vi "run_py.vi"(8 "error_in":errorcluster, 11 "preregistraion_data":T1) -> (0 "error_out":errorcluster)   [LabVIEW 2018]
uses:
  controls/preregistration_data.ctl
panel:
  out "mac_db.txt creation progress":i32(slide) scale=0.0..65535.0
  in  "stop":bool
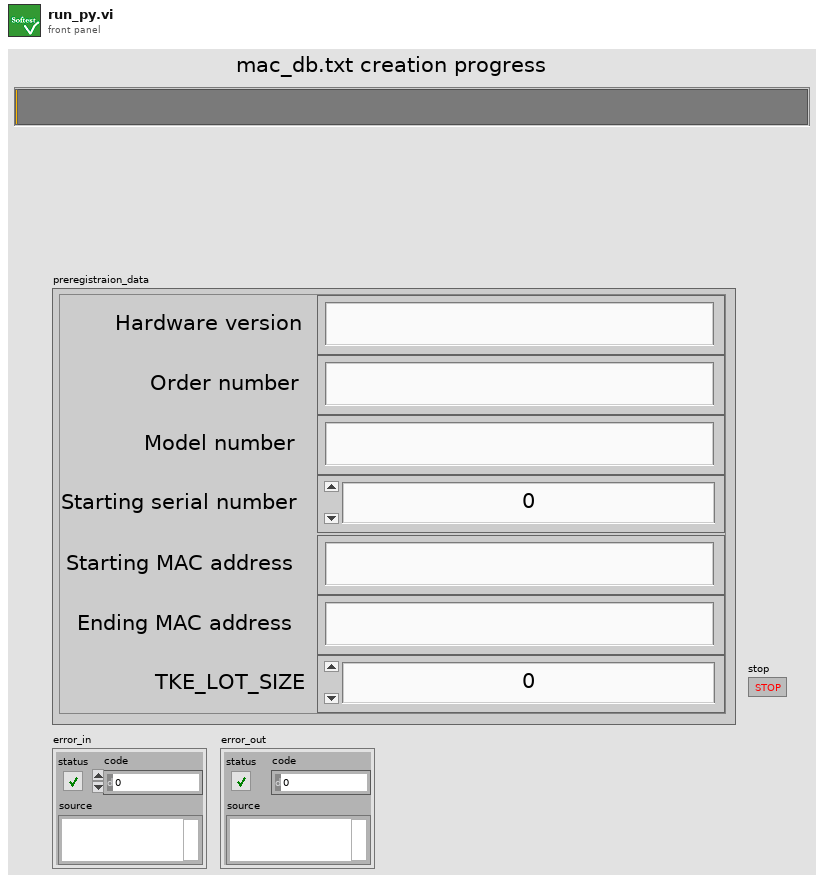
[diagram p1: front panel]
types:
  T1 = typedef "preregistration_data.ctl" = cluster{"Hardware version":string, "Order number":string, "Model number":string, "Starting serial number":i32, "Starting MAC address":string, "Ending MAC address":string, "TKE_LOT_SIZE":i32}
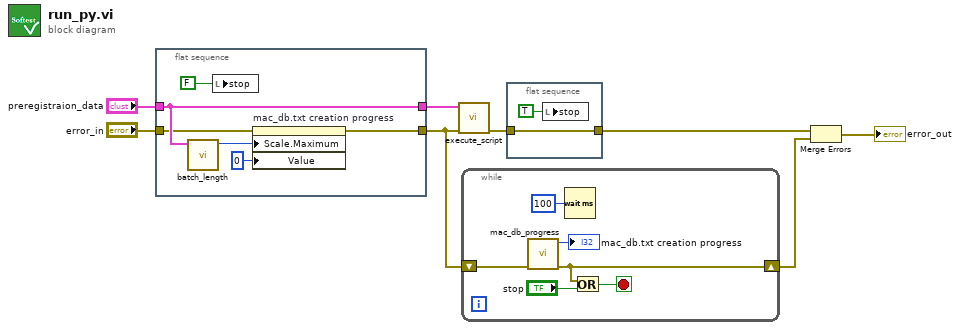
[diagram p0: block diagram]
diagram:
  n1 = flat-sequence {
    tunnel: [w13] -> w8
    tunnel: "preregistraion_data" -> [w13]
    tunnel: "error_in" -> [w11]
    tunnel: [w9] -> w4
    frame #0 {
      n2 = call "batch_length.vi"("preregistraion_data"=w13) -> ("batch_length"=w12:i32)  [unwired: 10 in]
      n3 = local write "stop"(FALSE) -> ()
      n4 = property on="mac_db.txt creation progress" class="Slide (strict)"(error in=w11, "Scale.Maximum"=w12, "Value"=0 ("mac_db.txt creation progress")) -> (error out=w9:errorcluster)  [unwired: 1 in, 1 out]
    }
  }
  n5 = call "execute_script.vi"("error in (no error)"=w4, "preregistraion_data"=w8) -> ("error out"=w7:errorcluster)  [unwired: 9 in]
  n6 = while {
    shift-right: [w15] -> w3
    shift-left: w4 -> [w16]
    stop <- w17 stop-if-true
    n7 = call "mac_db_progress.vi"("error in"=w16) -> ("error out"=w15:errorcluster, "mac_db_lines"=→"mac_db.txt creation progress":i32)  [unwired: 9 in]
    n8 = Wait (ms)(milliseconds to wait=u32 100) -> ()  [unwired: 1 out]
    n9 = Or(x=w15, y="stop") -> (x .or. y?=w17:bool)
  }
  n10 = flat-sequence {
    tunnel: [w22] -> w2
    tunnel: w7 -> [w22]
    frame #0 {
      n11 = local write "stop"(TRUE ("stop")) -> ()
    }
  }
  n12 = Merge Errors(w2, w3) -> (→"error_out":errorcluster)
